vi "Lock_Buttons.vi"(8 "Fehler (in)":errorcluster caption="Fehler", 10 "Disable Time":u32=1500, 11 "Bool Reference":T1) -> (0 "Fehler (out)":errorcluster caption="Fehler")   [LabVIEW 2013]
panel:
  out "Bool Ref":T1
  in  "exp cclock":bool
  in  "exp clock":bool
  in  "prep cclock":bool
  in  "prep clock":bool
  in  "down":bool
  in  "up":bool
  in  "right":bool
  in  "left":bool
  in  "out":bool
  in  "in":bool
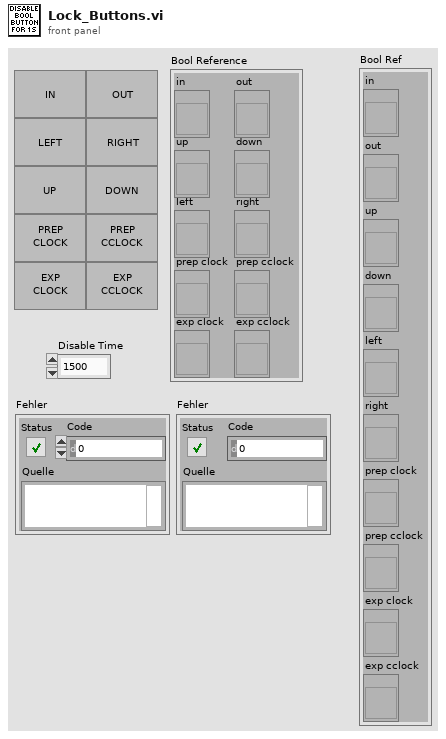
[diagram p1: front panel]
types:
  T1 = cluster{"in":refnum<vi>, "out":refnum<vi>, "up":refnum<vi>, "down":refnum<vi>, "left":refnum<vi>, "right":refnum<vi>, "prep clock":refnum<vi>, "prep cclock":refnum<vi>, "exp clock":refnum<vi>, "exp cclock":refnum<vi>}
  T2 = enum8{"Enabled", "Disabled", "Disabled and Grayed Out"}
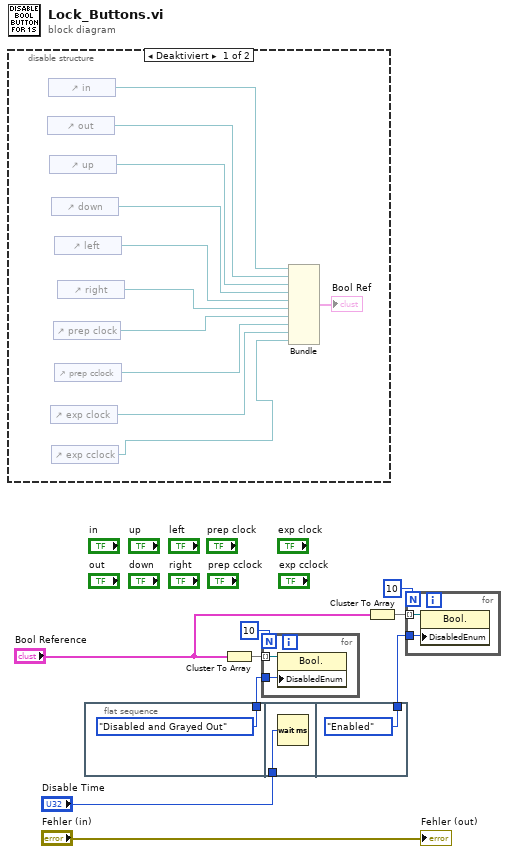
[diagram p0: block diagram]
diagram:
  n1 = disable-structure shown="Deaktiviert" {
    frame Disabled {
      n2 = control-ref of="out"() -> (w20:refnum<vi>)
      n3 = control-ref of="in"() -> (w11:refnum<vi>)
      n4 = control-ref of="up"() -> (w19:refnum<vi>)
      n5 = control-ref of="exp clock"() -> (w13:refnum<vi>)
      n6 = control-ref of="down"() -> (w18:refnum<vi>)
      n7 = control-ref of="exp cclock"() -> (w12:refnum<vi>)
      n8 = control-ref of="prep clock"() -> (w15:refnum<vi>)
      n9 = control-ref of="left"() -> (w17:refnum<vi>)
      n10 = control-ref of="prep cclock"() -> (w14:refnum<vi>)
      n11 = control-ref of="right"() -> (w16:refnum<vi>)
      n12 = Bundle("in"=w11, "out"=w20, "up"=w19, "down"=w18, "left"=w17, "right"=w16, "prep clock"=w15, "prep cclock"=w14, "exp clock"=w13, "exp cclock"=w12) -> (→"Bool Ref":T1)  [unwired: 1 in]
    }
    frame Enabled {
    }
  }
  n13 = flat-sequence {
    tunnel: [T2."Disabled and Grayed Out" ("Deaktiviert")] -> w8
    tunnel: "Disable Time" -> [w22]
    tunnel: [T2."Enabled" ("Deaktiviert")] -> w4
    frame #0 {
    }
    frame #1 {
      n14 = Wait (ms)(milliseconds to wait=w22) -> ()  [unwired: 1 out]
    }
    frame #2 {
    }
  }
  n15 = Cluster To Array(cluster="Bool Reference") -> (array=w9:refnum<vi>[])
  n16 = for {
    N: 10 -> [_]
    tunnel: w9 -> [w25] mode=indexing
    tunnel: w8 -> [w24]
    n17 = property on="Eigenschaftsknoten" class="Bool."(reference=w25, "DisabledEnum"=w24) -> ()  [unwired: 1 in, 2 out]
  }
  n18 = Cluster To Array(cluster="Bool Reference") -> (array=w6:refnum<vi>[])
  n19 = for {
    N: 10 -> [_]
    tunnel: w6 -> [w27] mode=indexing
    tunnel: w4 -> [w26]
    n20 = property on="Eigenschaftsknoten" class="Bool."(reference=w27, "DisabledEnum"=w26) -> ()  [unwired: 1 in, 2 out]
  }
  "Fehler (out)" <- "Fehler (in)"
